vi "2 Point Moving Average.vi"(11 "Peak Data":dbl[](array[numeric])) -> (2 "Smoothed Data":dbl[](array[numeric]), 3 "Orig VS Smoothed":cluster{dbl, dbl}[](array[cluster]))   [LabVIEW 2015]
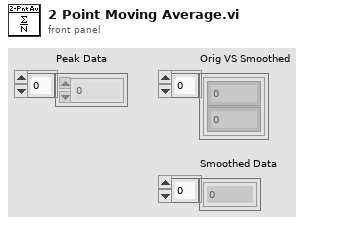
[diagram p1: front panel]
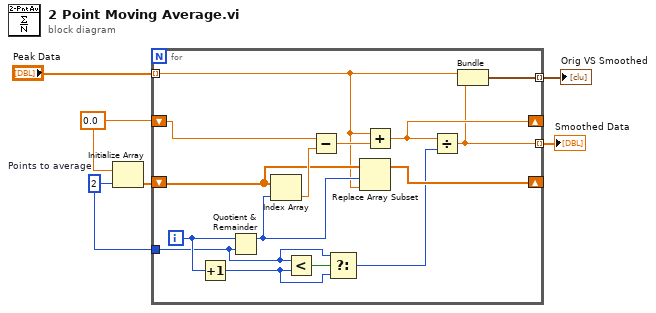
[diagram p0: block diagram]
diagram:
  w2 = 2  # Points to average
  w1 = 0.0 ("y")
  n1 = Initialize Array(w1, w2) -> (w3:dbl[])
  n2 = for {
    tunnel: w2 -> [w10]
    shift-left: w3 -> [w19]
    shift-right: [w21] -> _
    shift-left: w1 -> [w17]
    shift-right: [w15] -> _
    tunnel: "Peak Data" -> [w9] mode=indexing
    tunnel: [w8] -> w5 mode=indexing
    tunnel: [w7] -> w6 mode=indexing
    i -> [w14]
    n3 = Increment(x=w14) -> (x+1=w11:i32)
    n4 = Quotient & Remainder(x=w14, y=w10) -> (x-y*floor(x/y)=w16:i32)  [unwired: 1 out]
    n5 = Index Array(array=w19, index=w16) -> (element=w20:dbl)
    n6 = Less?(x=w10, y=w11) -> (x < y?=w13:bool)
    n7 = Subtract(x=w17, y=w20) -> (x-y=w18:dbl)
    n8 = Select(t=w10, s=w13, f=w11) -> (s? t:f=w12:i32)
    n9 = Replace Array Subset(array=w19, new element=w9, index=w16) -> (w21:dbl[])
    n10 = Add(x=w9, y=w18) -> (x+y=w15:dbl)
    n11 = Divide(x=w15, y=w12) -> (x/y=w8:dbl)
    n12 = Bundle(w9, w8) -> (w7:cluster{dbl, dbl})  [unwired: 1 in]
  }
  "Orig VS Smoothed" <- w6
  "Smoothed Data" <- w5
